vi "Read Linker Info.vi"(7 "Application Reference (Local Reference)":refnum<vi>, 8 "error in (no error)":errorcluster, 9 "polys & tds (T)":bool=TRUE, 10 "recursive? (F)":bool, 11 "paths to read":path[](array[path])) -> (0 "error out":errorcluster, 2 "Read Linker Info from File":T1(array[cluster]), 5 "dup Application Reference":refnum<vi>)   [LabVIEW 2011]
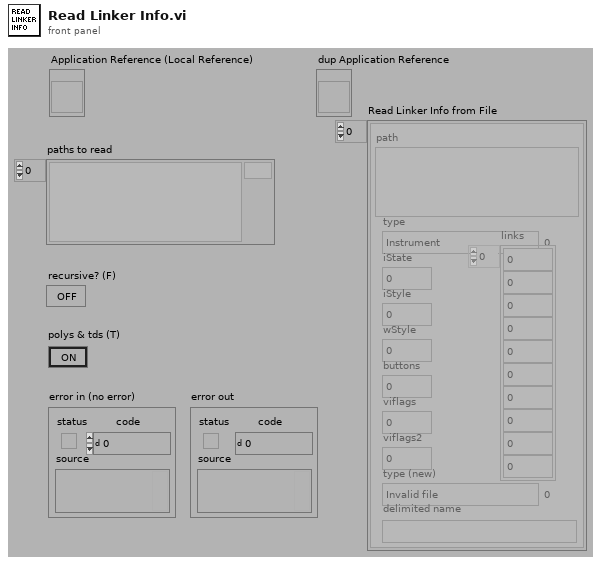
[diagram p1: front panel]
types:
  T1 = cluster{"path":path, "type":enum32{"Instrument", "Control", "CIN", "External subroutine", "Shared library", "Run-time menu", "Help file", "Palette menu", "Polymorphic VI", "Library", "Library (10)"}, "iState":u32, "iStyle":u16, "wStyle":u16, "buttons":u16, "viflags":u32, "viflags2":u32, "links":u32[], "type (new)":enum32{"Invalid file", "Unknown type", "Instrument", "Control", "Polymorphic VI", "Project", "Library", "LVClass", "XControl", "XNode", "Shared library", ".NET assembly", "ActiveX interface", "CIN", "Run-time menu", "Palette menu", "Help file", "LLB", "XNode Edit Dependency", "Class Private Data Control", "Statechart", "MathScript .m file"}, "delimited name":string}[]
  T2 = cluster{"path":path, "type":enum32{"Instrument", "Control", "CIN", "External subroutine", "Shared library", "Run-time menu", "Help file", "Palette menu", "Polymorphic VI", "Library", "Library (10)"}, "iState":u32, "iStyle":u16, "wStyle":u16, "buttons":u16, "viflags":u32, "viflags2":u32, "links":u32[], "type (new)":enum32{"Invalid file", "Unknown type", "Instrument", "Control", "Polymorphic VI", "Project", "Library", "LVClass", "XControl", "XNode", "Shared library", ".NET assembly", "ActiveX interface", "CIN", "Run-time menu", "Palette menu", "Help file", "LLB", "XNode Edit Dependency", "Class Private Data Control", "Statechart", "MathScript .m file"}, "delimited name":string}
  T3 = enum32{"Include all", "Run time only", "Run time only (No typedefs & polys)"}
  T4 = enum32{"Invalid file", "Unknown type", "Instrument", "Control", "Polymorphic VI", "Project", "Library", "LVClass", "XControl", "XNode", "Shared library", ".NET assembly", "ActiveX interface", "CIN", "Run-time menu", "Palette menu", "Help file", "LLB", "XNode Edit Dependency", "Class Private Data Control", "Statechart", "MathScript .m file"}
  T5 = enum32{"Instrument", "Control", "CIN", "External subroutine", "Shared library", "Run-time menu", "Help file", "Palette menu", "Polymorphic VI", "Library", "Library (10)"}
  T6 = typedef "NI_FileType.lvlib/LVFileType.ctl" = enum32{"Invalid file", "Unknown type", "Instrument", "Control", "Polymorphic VI", "Project", "Library", "LVClass", "XControl", "XNode", "Shared library", ".NET assembly", "ActiveX interface", "CIN", "Run-time menu", "Palette menu", "Help file", "LLB", "XNode Edit Dependency", "Class Private Data Control", "Statechart", "MathScript .m file", "Ladder Diagram", "LVLibp"}
  T7 = cluster{"path":path, "delimited name":string, "type":T6, "iState":u32, "iStyle":u16, "wStyle":u16, "buttons":u16, "viflags":u32, "viflags2":u32, "links":u32[]}[]
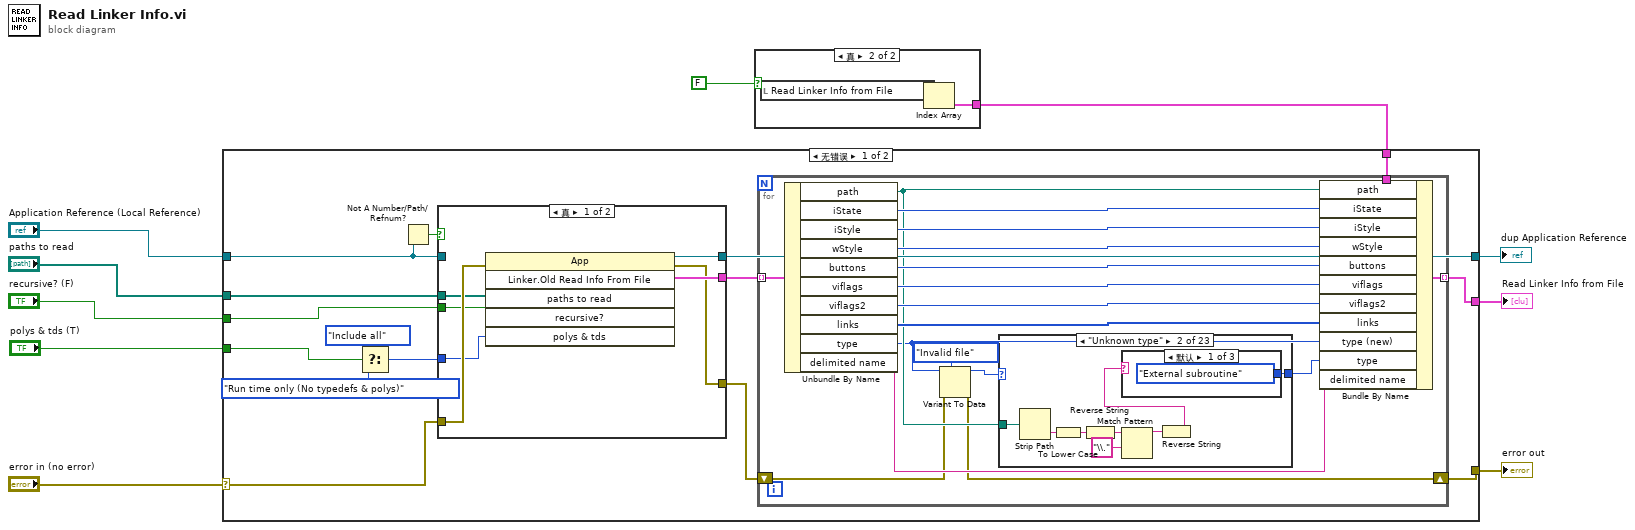
[diagram p0: block diagram]
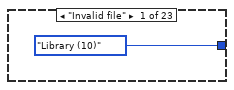
[diagram p3: hidden frame]
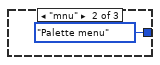
[diagram p4: hidden frame]
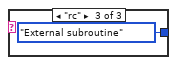
[diagram p5: hidden frame]
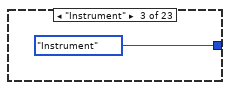
[diagram p6: hidden frame]
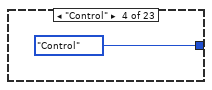
[diagram p7: hidden frame]
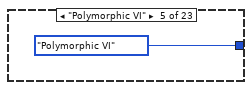
[diagram p8: hidden frame]
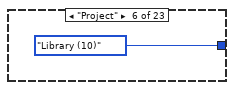
[diagram p9: hidden frame]
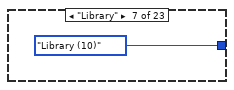
[diagram p10: hidden frame]
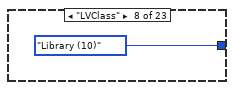
[diagram p11: hidden frame]
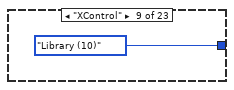
[diagram p12: hidden frame]
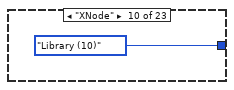
[diagram p13: hidden frame]
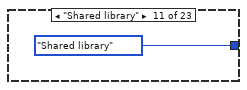
[diagram p14: hidden frame]
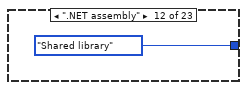
[diagram p15: hidden frame]
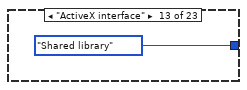
[diagram p16: hidden frame]
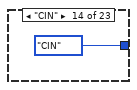
[diagram p17: hidden frame]
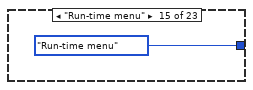
[diagram p18: hidden frame]
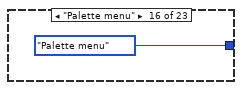
[diagram p19: hidden frame]
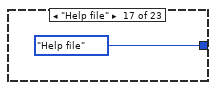
[diagram p20: hidden frame]
diagram:
  n1 = case shown="真" FALSE {
    tunnel: [_ w11] -> w2
    frame False {
    }
    frame True {
      n2 = local read "Read Linker Info from File"() -> (w12:T1)
      n3 = Index Array(array=w12) -> (element=w11:T2)  [unwired: 1 in]
    }
  }
  n4 = case shown="无错误" "error in (no error)" {
    selector: "error in (no error)" -> [w27 w95]
    tunnel: [w21 w95] -> w3
    tunnel: "paths to read" -> [w25 _]
    tunnel: "recursive? (F)" -> [w24 _]
    tunnel: "Application Reference (Local Reference)" -> [w23 w94]
    tunnel: [w26 w94] -> w7
    tunnel: [w22 _] -> w4
    tunnel: "polys & tds (T)" -> [w17 _]
    tunnel: w2 -> [w13 _]
    frame No Error {
      n5 = Select(t=T3."Include all" ("Links To Include"), s=w17, f=T3."Run time only (No typedefs & polys)" ("Links To Include")) -> (s? t:f=w14:T3)
      n6 = Not A Number/Path/Refnum?(number/path/refnum=w23) -> (NaN/Path/Refnum?=w20:bool)
      n7 = case shown="真" w20 {
        tunnel: w27 -> [w85 w93]
        tunnel: [w84 w92] -> w26
        tunnel: [w83 w91] -> w19
        tunnel: w25 -> [w82 w90]
        tunnel: w24 -> [w81 w89]
        tunnel: [w80 w88] -> w18
        tunnel: w23 -> [_ w87]
        tunnel: w14 -> [w79 w86]
        frame True {
          n8 = invoke class="App" method="Linker.Old Read Info From File"(error in=w85, "paths to read"=w82, "recursive?"=w81, "polys & tds"=w79) -> (reference out=w84:refnum<vi>, error out=w80:errorcluster, "Linker:Read Info From File"=w83:T7)  [unwired: 2 in, 3 out]
        }
        frame False {
          n9 = invoke class="App" method="Linker.Old Read Info From File"(reference=w87, error in=w93, "paths to read"=w90, "recursive?"=w89, "polys & tds"=w86) -> (reference out=w92:refnum<vi>, error out=w88:errorcluster, "Linker:Read Info From File"=w91:T7)  [unwired: 1 in, 3 out]
        }
      }
      n10 = for {
        tunnel: w19 -> [w45] mode=indexing
        tunnel: [w35] -> w22 mode=indexing
        shift-right: [w28] -> w21
        shift-left: w18 -> [w29]
        tunnel: w13 -> [w44]
        n11 = Unbundle By Name(w45) -> ("path"=w33:path, "iState"=w43:u32, "iStyle"=w42:u16, "wStyle"=w41:u16, "buttons"=w40:u16, "viflags"=w39:u32, "viflags2"=w38:u32, "links"=w37:u32[], "type"=w31:T6, "delimited name"=w34:string)
        n12 = Variant To Data(error in=w29, type=T4."Invalid file" ("type (new)"), Variant=w31) -> (data=w30:T4, error out=w28:errorcluster)
        n13 = case shown="\"Unknown type\"" w30 {
          tunnel: [T5."Library (10)" ("type") w54 T5."Instrument" ("type") T5."Control" ("type") T5."Polymorphic VI" ("type") T5."Library (10)" ("type") T5."Library (10)" ("type") T5."Library (10)" ("type") T5."Library (10)" ("type") T5."Library (10)" ("type") T5."Shared library" ("type") T5."Shared library" ("type") T5."Shared library" ("type") T5."CIN" ("type") T5."Run-time menu" ("type") T5."Palette menu" ("type") T5."Help file" ("type") T5."Library" ("type") T5."External subroutine" ("type") T5."Control" ("type") T5."External subroutine" ("type") T5."External subroutine" ("type") T5."Library (10)" ("type")] -> w36
          tunnel: w33 -> [_ w53 _ _ _ _ _ _ _ _ _ _ _ _ _ _ _ _ _ _ _ _ _]
          frame "Invalid file" {
          }
          frame "Unknown type" {
            n14 = Strip Path(path=w53) -> (name=w52:string)  [unwired: 1 out]
            n15 = To Lower Case(string=w52) -> (all lower case string=w51:string)
            n16 = Reverse String(1:w51) -> (0:w50:string)
            n17 = Match Pattern(string=w50, regular expression="\\.") -> (before substring=w48:string)  [unwired: 1 in, 3 out]
            n18 = Reverse String(1:w48) -> (0:w47:string)
            n19 = case shown="默认" w47 {
              tunnel: [T5."External subroutine" ("type") T5."Palette menu" ("type") T5."External subroutine" ("type")] -> w54
              frame Default {
              }
              frame "mnu" {
              }
              frame "rc" {
              }
            }
          }
          frame "Instrument" {
          }
          frame "Control" {
          }
          frame "Polymorphic VI" {
          }
          frame "Project" {
          }
          frame "Library" {
          }
          frame "LVClass" {
          }
          frame "XControl" {
          }
          frame "XNode" {
          }
          frame "Shared library" {
          }
          frame ".NET assembly" {
          }
          frame "ActiveX interface" {
          }
          frame "CIN" {
          }
          frame "Run-time menu" {
          }
          frame "Palette menu" {
          }
          frame "Help file" {
          }
          frame "LLB" {
          }
          frame "XNode Edit Dependency" {
          }
          frame "Class Private Data Control" {
          }
          frame "Statechart" {
          }
          frame "MathScript .m file" {
          }
          frame Default {
          }
        }
        n20 = Bundle By Name(cluster=w44, "path"=w33, "iState"=w43, "iStyle"=w42, "wStyle"=w41, "buttons"=w40, "viflags"=w39, "viflags2"=w38, "links"=w37, "type (new)"=w31, "type"=w36, "delimited name"=w34) -> (w35:T2)
      }
    }
    frame Error {
    }
  }
  "Read Linker Info from File" <- w4
  "error out" <- w3
  "dup Application Reference" <- w7
